vi "FP Ref Testing.vi"() -> ()   [LabVIEW 2018]
panel:
  out "Array":T1(array[cluster])
  in  "LabVIEW Object":refnum<class>
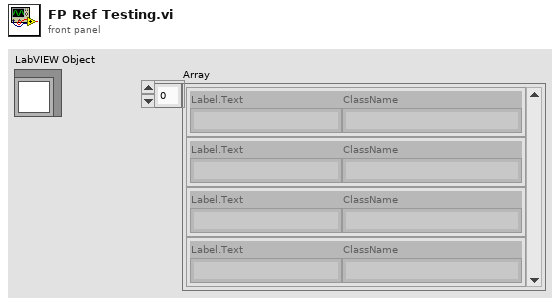
[diagram p1: front panel]
types:
  T1 = cluster{"Label.Text":string, "ClassName":string}[]
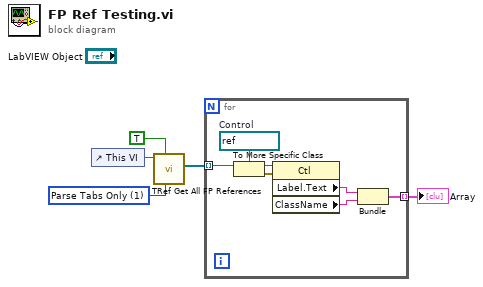
[diagram p0: block diagram]
diagram:
  w4 = u16 1 items=["Parse All", "Parse Tabs Only"] ("Parsing Rule")
  n1 = control-ref of="This VI"() -> (w2:refnum<vi>)
  n2 = call <vilib>:"TRef Get All FP References.vi"("Parsing Rule"=w4, "Ignore Decorations?"=TRUE, "VI Refnum"=w2) -> ("All FP Objects"=w3:refnum<vi>[])  [unwired: 4 in, 4 out]
  n3 = for {
    tunnel: w3 -> [w11] mode=indexing
    tunnel: [w6] -> w1 mode=indexing
    w12 = refnum<vi> refnum  # Control
    n4 = To More Specific Class(target class=w12, reference=w11) -> (specific class reference=w10:refnum<vi>, error out=w9:errorcluster)  [unwired: 1 in]
    n5 = property class="Ctl"(reference=w10, error in=w9) -> ("Label.Text"=w8:string, "ClassName"=w7:string)  [unwired: 2 out]
    n6 = Bundle("Label.Text"=w8, "ClassName"=w7) -> (w6:cluster{"Label.Text":string, "ClassName":string})  [unwired: 1 in]
  }
  "Array" <- w1
